vi "saveDataNodeBegin.vi"(8 "error in (no error)":errorcluster, 9 "indent":i32, 10 "XML Refnum in":refnum<file>, 11 "Void in":refnum<class "Void.lvclass">) -> (0 "error out":errorcluster, 2 "XML Refnum out":refnum<file>, 3 "Chennel out":refnum<class "Void.lvclass">)   [LabVIEW 2013, in "Void.lvclass"]
doc: "Begins the process of saving a xceData Node to an XML formatted file."
uses:
  Void.lvclass
  xCE/xceNode/xceNode.lvclass
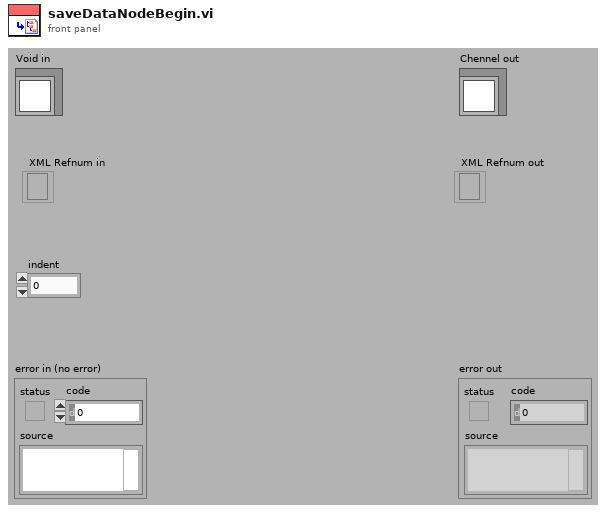
[diagram p1: front panel]
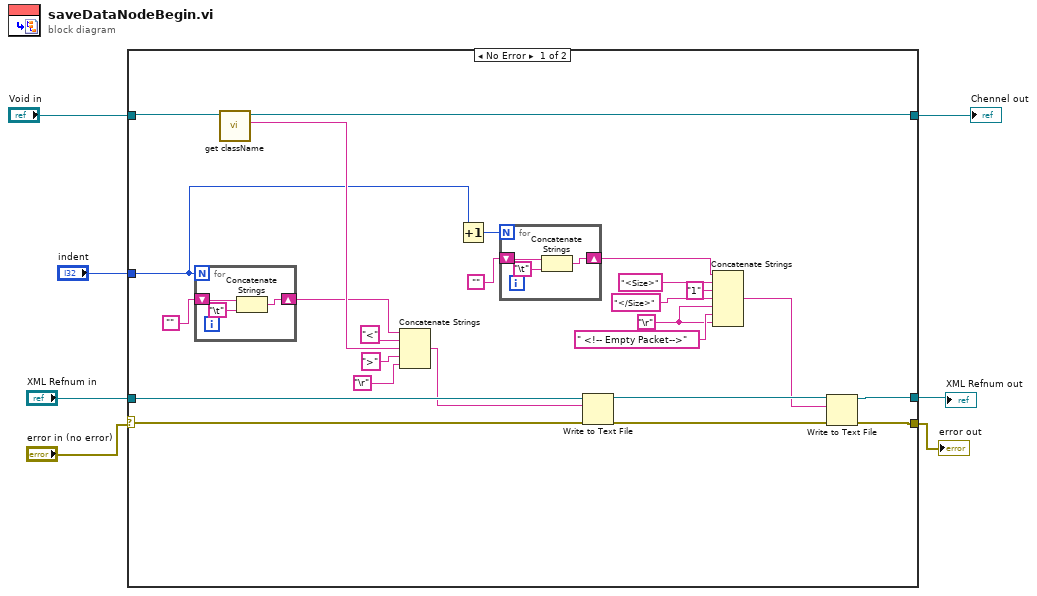
[diagram p0: block diagram]
diagram:
  n1 = case shown="No Error" "error in (no error)" {
    selector: "error in (no error)" -> [w30 w40]
    tunnel: "Void in" -> [w24 w41]
    tunnel: [w13 w41] -> w6
    tunnel: [w12 w40] -> w1
    tunnel: [w14 w39] -> w2
    tunnel: "indent" -> [w10 _]
    tunnel: "XML Refnum in" -> [w31 w39]
    frame No Error {
      w8 = "\r"
      n2 = for {
        N: w10 -> [_]
        shift-right: [w36] -> w19
        shift-left: "" -> [w38]
        n3 = Concatenate Strings(w38, "\t") -> (w36:string)
      }
      n4 = call "get className.vi"("xceNode in"=w24) -> ("Class name"=w20:string, "xceNode out"=w13:refnum<class "Void.lvclass">)  [unwired: 8 in, 1 out]
      n5 = Concatenate Strings(w19, "<", w20, ">", "\r") -> (w18:string)
      n6 = Increment(x=w10) -> (x+1=w17:i32)
      n7 = for {
        N: w17 -> [_]
        shift-right: [w33] -> w15
        shift-left: "" -> [w35]
        n8 = Concatenate Strings(w35, "\t") -> (w33:string)
      }
      n9 = Write to Text File(file (use dialog)=w31, text=w18, error in=w30) -> (refnum out=w29:refnum<file>, error out=w25:errorcluster)  [unwired: 1 in, 1 out]
      n10 = Concatenate Strings(w15, "<Size>" ("string"), "1" ("string"), "</Size>" ("string"), w8, " <!-- Empty Packet-->" ("string"), w8) -> (w26:string)
      n11 = Write to Text File(file (use dialog)=w29, text=w26, error in=w25) -> (refnum out=w14:refnum<file>, error out=w12:errorcluster)  [unwired: 1 in, 1 out]
    }
    frame Error {
    }
  }
  "error out" <- w1
  "Chennel out" <- w6
  "XML Refnum out" <- w2
